vi "CreateCurveNamesvb.vi"(8 "error in":errorcluster, 9 "NomDon":string[](array[string])=["RTêta;", "X&Y;"], 10 "IndCourbe":i64 caption="Numéro de Balayage", 11 "Experiment.lvclass In":refnum<class "Experiment.lvclass">) -> (0 "error out":errorcluster, 2 "Scan list":string[](array[string]), 3 "Experiment.lvclass Out":refnum<class "Experiment.lvclass">, 4 "ScanTableSize":i32[](array[numeric]))   [LabVIEW 2019, in "Experiment.lvclass"]
doc: "Ce Vi créer la ligne d'entête du fichier texte de sauvegarde à partir du nombre de courbe voulu."
uses:
  Experiment.lvclass
  Experiment.lvclass/Experiment.ctl
  Calculations Class/Calculations.lvclass
  Calculations Class/Calculations.lvclass/Calculations.ctl
  Calculations Class/Accessor/GetCalcEveryScanPar.vi
  DevicesClass/BaseDevice/BaseDevice.lvclass
panel:
  out "CalcNameInd":i32[](array[numeric])
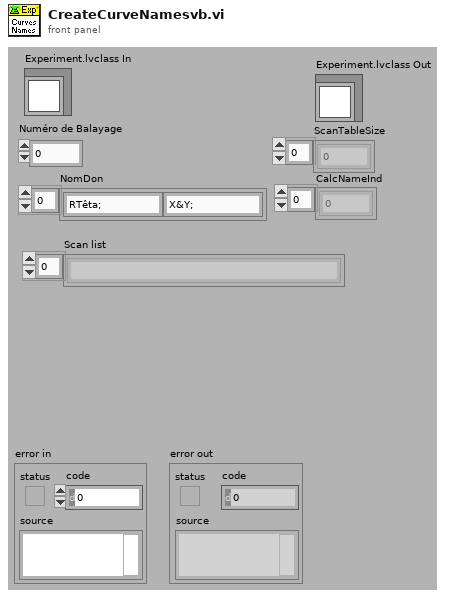
[diagram p1: front panel]
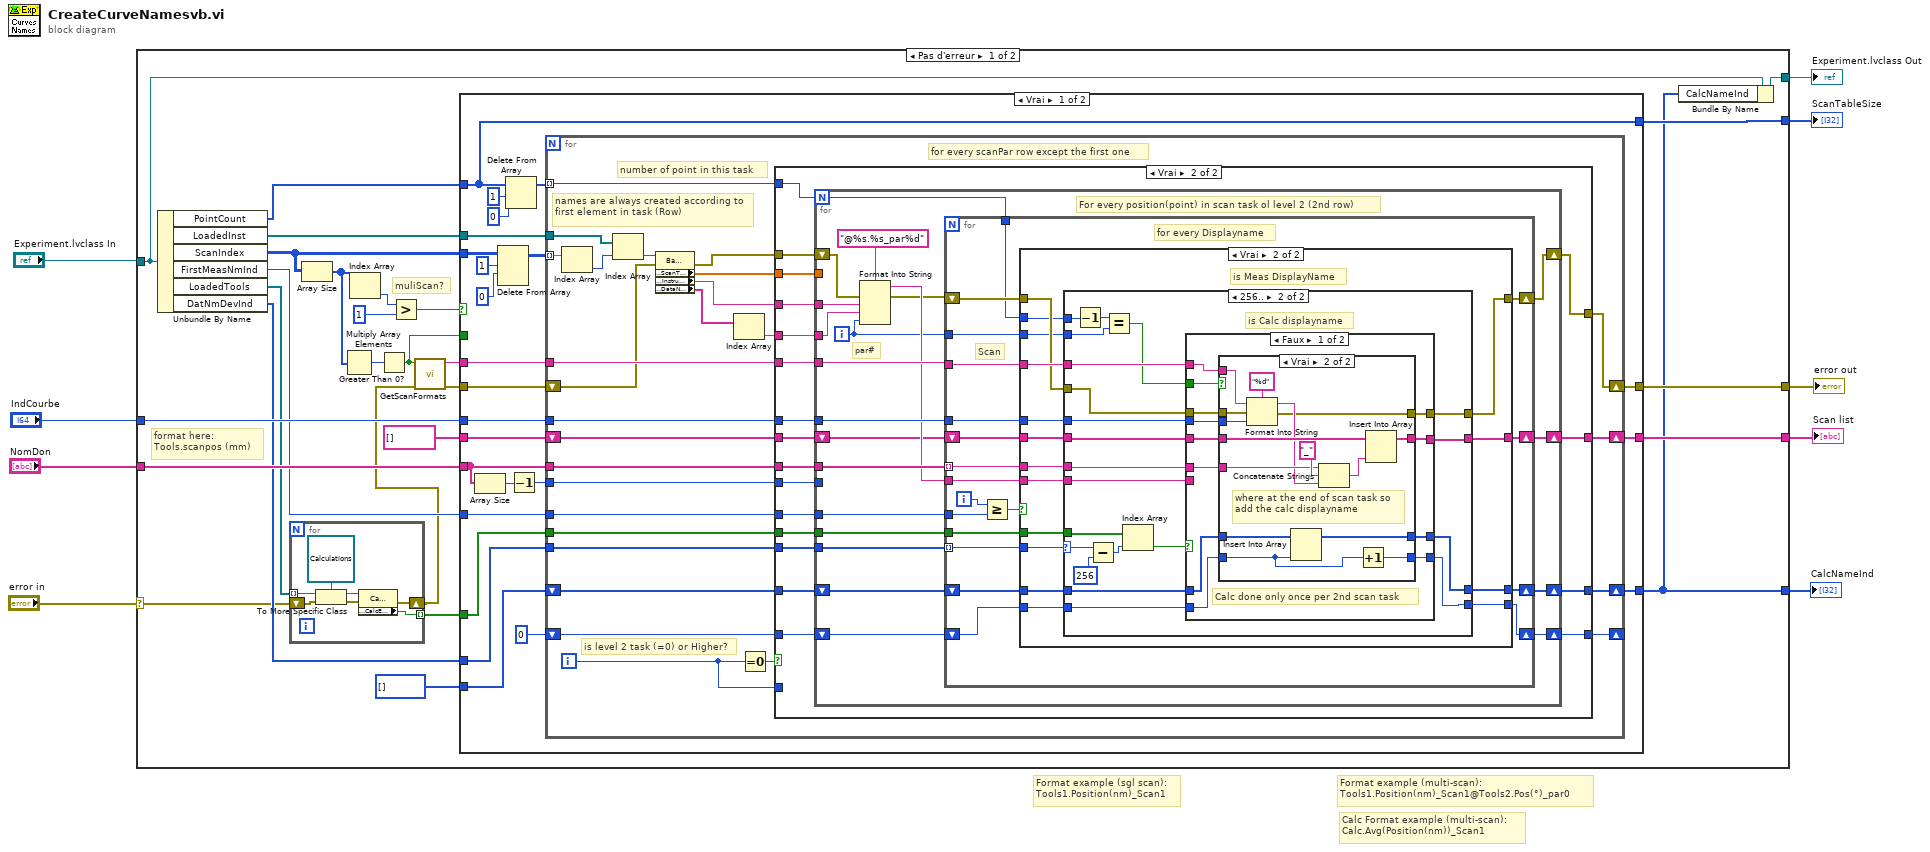
[diagram p0: block diagram]
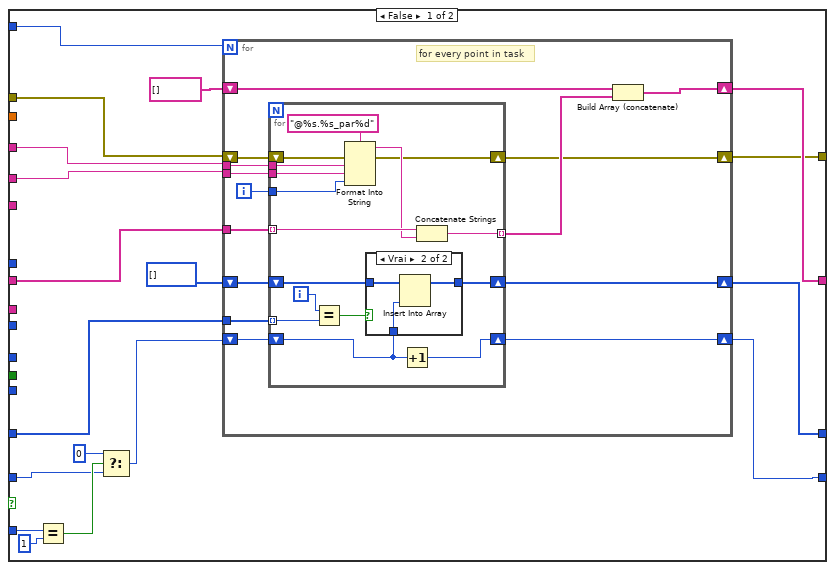
[diagram p2: hidden frame]
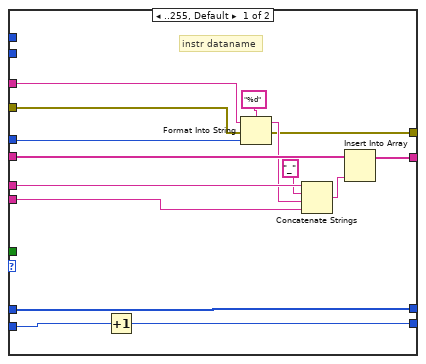
[diagram p5: hidden frame]
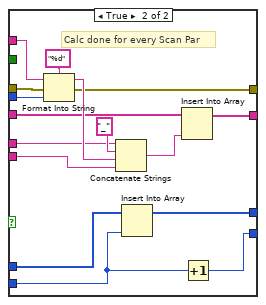
[diagram p7: hidden frame]
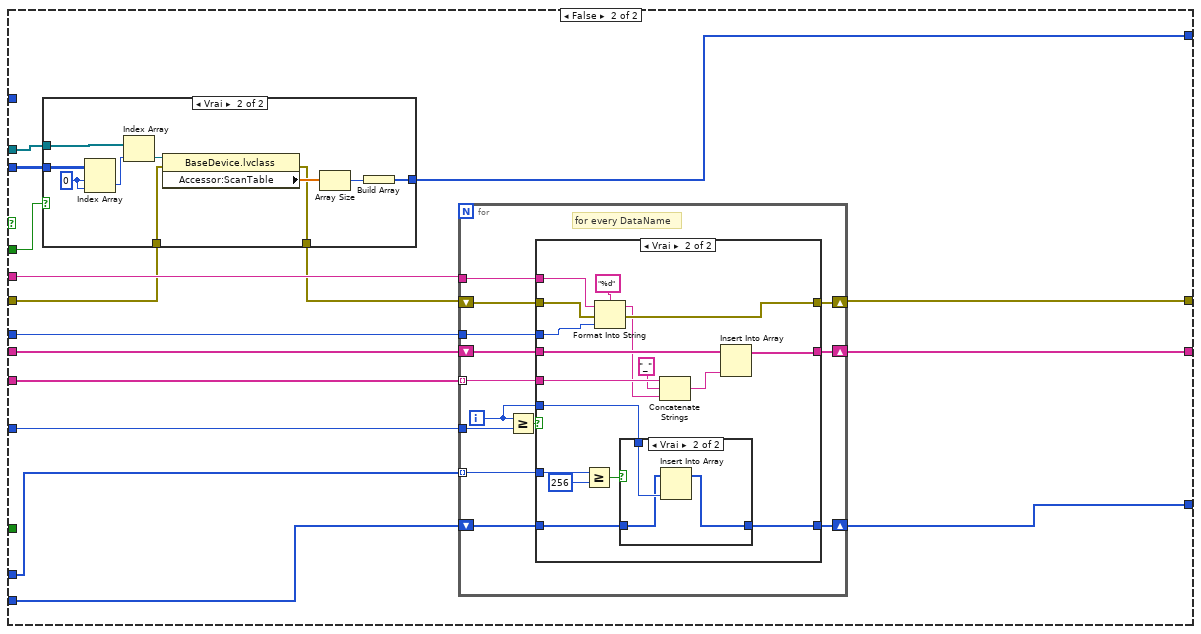
[diagram p8: hidden frame]
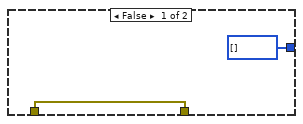
[diagram p9: hidden frame]
diagram:
  # "Calc Format example (multi-scan):\nCalc.Avg(Position(nm))_Scan1"
  # "Format example (multi-scan):\nTools1.Position(nm)_Scan1@Tools2.Pos(°)_par0"
  # "Format example (sgl scan):\nTools1.Position(nm)_Scan1"
  n1 = case shown="Pas d'erreur" "error in" {
    selector: "error in" -> [w15 w375]
    tunnel: [w26 w375] -> w8
    tunnel: [w32 _] -> w7
    tunnel: "NomDon" -> [w33 _]
    tunnel: "Experiment.lvclass In" -> [w23 w374]
    tunnel: "IndCourbe" -> [w35 _]
    tunnel: [w11 w374] -> w3
    tunnel: [w22 _] -> w2
    tunnel: [w10 _] -> w1
    frame No Error {
      # "format here:\nTools.scanpos (mm)"
      # "muliScan?"
      n2 = Unbundle By Name(w23) -> ("PointCount"=w18:i32[], "LoadedInst"=w27:refnum<class "BaseDevice.lvclass">[], "ScanIndex"=w28:i32[][], "FirstMeasNmInd"=w25:i32, "LoadedTools"=w16:refnum<class "BaseDevice.lvclass">[], "DatNmDevInd"=w17:i32[])
      n3 = for {
        tunnel: w16 -> [w40] mode=indexing
        shift-right: [w38] -> w14
        shift-left: w15 -> [w39]
        tunnel: [w37] -> w13 mode=indexing
        n4 = To More Specific Class(target class=refnum<class "Calculations.lvclass"> refnum ("Calculations.lvclass"), reference=w40, error in=w39) -> (specific class reference=w42:refnum<class "Calculations.lvclass">, error out=w43:errorcluster)
        n5 = property class="Calculations.lvclass"(reference=w42, error in=w43) -> (error out=w38:errorcluster, "Accessor:CalcEveryScanPar"=w37:bool)  [unwired: 1 out]
      }
      n6 = Array Size(array=w28) -> (size(s)=w20:i32[])
      n7 = Multiply Array Elements(1:w20) -> (0:w30:i32)
      n8 = Index Array(array=w20) -> (element=w19:i32)  [unwired: 1 in]
      n9 = Greater Than 0?(x=w30) -> (x > 0?=w21:bool)
      n10 = Greater?(x=w19, y=1) -> (0:w24:bool)
      n11 = call "GetScanFormats.vi"("ErrorIn(No Error)"=w14, "Scan(T)"=w21) -> ("sortie d'erreur"=w34:errorcluster, "Prefixe"=w36:string)  [unwired: 7 in, 1 out]
      n12 = case shown="Vrai" w24 {
        tunnel: w36 -> [w67 w324]
        tunnel: w35 -> [w66 w323]
        tunnel: w34 -> [w65 w314]
        tunnel: w33 -> [w51 w322]
        tunnel: [w60 w321] -> w32
        tunnel: string[] [] -> [w52 w320]
        tunnel: w28 -> [w64 w317]
        tunnel: w27 -> [w63 w316]
        tunnel: [w62 w319] -> w26
        tunnel: w25 -> [w61 w318]
        tunnel: [w47 w315] -> w22
        tunnel: w21 -> [_ w312]
        tunnel: w18 -> [w47 _]
        tunnel: w17 -> [w53 w310]
        tunnel: w13 -> [w48 _]
        tunnel: i32[] [] ("DatNameInd") -> [w46 w311]
        tunnel: [w44 w309] -> w10
        frame True {
          n13 = Array Size(array=w51) -> (size(s)=w50:i32)
          n14 = Delete From Array(array=w64, length=1 ("longueur"), index (row)=0 ("indice (ligne)")) -> (array with subset deleted=w59:i32[][])  [unwired: 1 in, 1 out]
          n15 = Delete From Array(array=w47, length=1 ("longueur"), index=0 ("indice")) -> (array with subset deleted=w55:i32[])  [unwired: 1 out]
          n16 = Decrement(x=w50) -> (x-1=w49:i32)
          n17 = for {
            tunnel: w67 -> [w94]
            tunnel: w66 -> [w93]
            tunnel: w51 -> [w92]
            tunnel: w59 -> [w91] mode=indexing
            tunnel: w63 -> [w90]
            shift-right: [w88] -> w62
            shift-left: w65 -> [w89]
            tunnel: w61 -> [w87]
            shift-right: [w84] -> w60
            shift-left: w52 -> [w83]
            tunnel: w55 -> [w82] mode=indexing
            tunnel: w53 -> [w75]
            tunnel: w48 -> [w74]
            tunnel: w49 -> [w73]
            shift-right: [w70] -> _
            shift-left: 0 ("Numérique") -> [w71]
            shift-right: [w69] -> w44
            shift-left: w46 -> [w72]
            i -> [w68]
            # "is level 2 task (=0) or Higher?"
            # "number of point in this task"
            # "names are always created according to first element in task (Row)"
            # "for every scanPar row except the first one"
            n18 = Index Array(array=w91) -> (element=w80:i32)  [unwired: 1 in]
            n19 = Index Array(array=w90, index=w80) -> (element=w79:refnum<class "BaseDevice.lvclass">)
            n20 = property class="BaseDevice.lvclass"(reference=w79, error in=w89) -> (error out=w81:errorcluster, "Accessor:ScanTable"=w77:dbl[], "Accessor:InstrumentName"=w85:string, "Accessor:DataNames"=w78:string[])  [unwired: 1 out]
            n21 = Index Array(array=w78) -> (element=w86:string)  [unwired: 1 in]
            n22 = Equal To 0?(x=w68) -> (x = 0?=w76:bool)
            n23 = case shown="Vrai" w76 {
              tunnel: w94 -> [_ w165]
              tunnel: w93 -> [_ w164]
              tunnel: w92 -> [_ w163]
              tunnel: [w107 w162] -> w88
              tunnel: w87 -> [_ w161]
              tunnel: w86 -> [w111 w160]
              tunnel: w85 -> [w112 w159]
              tunnel: [w108 w158] -> w84
              tunnel: w83 -> [w109 w157]
              tunnel: w82 -> [w105 w152]
              tunnel: w81 -> [w110 w156]
              tunnel: w77 -> [_ w155]
              tunnel: w75 -> [_ w154]
              tunnel: w74 -> [_ w153]
              tunnel: w73 -> [_ w151]
              tunnel: w72 -> [w101 w150]
              tunnel: w71 -> [w96 w149]
              tunnel: [w104 w148] -> w70
              tunnel: [w99 w147] -> w69
              tunnel: w68 -> [w103 _]
              frame False {
                n24 = Equal?(x=w103, y=1) -> (x = y?=w97:bool)
                n25 = Select(t=0, s=w97, f=w96) -> (s? t:f=w98:i32)
                n26 = for {
                  N: w105 -> [_]
                  tunnel: w112 -> [w126]
                  tunnel: w111 -> [w125]
                  shift-right: [w120] -> w107
                  shift-left: w110 -> [w124]
                  tunnel: w109 -> [w123]
                  shift-right: [w119] -> w108
                  shift-left: string[] [] -> [w118]
                  shift-right: [w117] -> w104
                  shift-left: w98 -> [w116]
                  tunnel: w101 -> [w115]
                  shift-right: [w113] -> w99
                  shift-left: i32[] [] ("DatNameInd") -> [w114]
                  i -> [w122]
                  # "for every point in task"
                  n27 = for {
                    tunnel: w126 -> [w141]
                    tunnel: w125 -> [w140]
                    tunnel: w123 -> [w138] mode=indexing
                    tunnel: w122 -> [w136]
                    tunnel: [w135] -> w121 mode=indexing
                    shift-right: [w134] -> w120
                    shift-left: w124 -> [w139]
                    shift-right: [w133] -> w117
                    shift-left: w116 -> [w127]
                    tunnel: w115 -> [w131] mode=indexing
                    shift-right: [w128] -> w113
                    shift-left: w114 -> [w129]
                    i -> [w130]
                    n28 = Equal?(x=w130, y=w131) -> (x = y?=w132:bool)
                    n29 = Format Into String(format string="@%s.%s_par%d" ("chaîne de format"), error in=w139, w141, w140, w136) -> (resulting string=w137:string, error out=w134:errorcluster)  [unwired: 1 in]
                    n30 = case shown="Vrai" w132 {
                      tunnel: w129 -> [w143 w146]
                      tunnel: [w143 w145] -> w128
                      tunnel: w127 -> [_ w144]
                      frame False {
                      }
                      frame True {
                        n31 = Insert Into Array(array=w146, new element=w144) -> (w145:i32[])  [unwired: 1 in]
                      }
                    }
                    n32 = Increment(x=w127) -> (x+1=w133:i32)
                    n33 = Concatenate Strings(w138, w137) -> (w135:string)
                  }
                  n34 = Build Array (concatenate)(w118, w121) -> (w119:string[])
                }
              }
              frame True {
                n35 = for {
                  N: w152 -> [w173]
                  tunnel: w165 -> [w186]
                  tunnel: w164 -> [w185]
                  tunnel: w163 -> [w184]
                  shift-right: [w170] -> w162
                  shift-left: w156 -> [w182]
                  tunnel: w161 -> [w183]
                  tunnel: w160 -> [w181]
                  tunnel: w159 -> [w180]
                  shift-right: [w171] -> w158
                  shift-left: w157 -> [w178]
                  tunnel: w155 -> [_]
                  tunnel: w154 -> [w175]
                  tunnel: w153 -> [w174]
                  tunnel: w151 -> [_]
                  shift-right: [w166] -> w147
                  shift-left: w150 -> [w169]
                  shift-right: [w167] -> w148
                  shift-left: w149 -> [w168]
                  i -> [w172]
                  # "par#"
                  # "For every position(point) in scan task ol level 2 (2nd row)"
                  n36 = Format Into String(format string="@%s.%s_par%d" ("chaîne de format"), error in=w182, w180, w181, w172) -> (resulting string=w179:string, error out=w177:errorcluster)  [unwired: 1 in]
                  n37 = for {
                    tunnel: w186 -> [w200]
                    tunnel: w184 -> [w203] mode=indexing
                    shift-right: [w204] -> w171
                    shift-left: w178 -> [w205]
                    tunnel: w185 -> [w201]
                    shift-right: [w191] -> w170
                    shift-left: w177 -> [w199]
                    tunnel: w183 -> [w198]
                    tunnel: w179 -> [w197]
                    tunnel: w175 -> [w196] mode=indexing
                    tunnel: w174 -> [w195]
                    tunnel: w173 -> [w193]
                    tunnel: w172 -> [w192]
                    shift-right: [w188] -> w166
                    shift-left: w169 -> [w189]
                    shift-right: [w187] -> w167
                    shift-left: w168 -> [w190]
                    i -> [w194]
                    # "Scan"
                    # "for every Displayname"
                    n38 = Greater Or Equal?(x=w194, y=w198) -> (x >= y?=w202:bool)
                    n39 = case shown="Vrai" w202 {
                      tunnel: w205 -> [w209 w225]
                      tunnel: [w209 w224] -> w204
                      tunnel: w203 -> [_ w223]
                      tunnel: w201 -> [_ w219]
                      tunnel: w200 -> [_ w222]
                      tunnel: w199 -> [w208 w221]
                      tunnel: w197 -> [_ w220]
                      tunnel: w196 -> [_ w217]
                      tunnel: w195 -> [_ w218]
                      tunnel: w193 -> [_ w216]
                      tunnel: w192 -> [_ w215]
                      tunnel: [w208 w214] -> w191
                      tunnel: w190 -> [w206 w213]
                      tunnel: w189 -> [w207 w212]
                      tunnel: [w207 w211] -> w188
                      tunnel: [w206 w210] -> w187
                      frame False {
                        # "in a scan the first items are the scanpar (var param): dont include it in graph legend"
                      }
                      frame True {
                        # "is Meas DisplayName"
                        n40 = case shown="256.." w217 {
                          selector: w217 -> [_ w252]
                          tunnel: w225 -> [w240 w258]
                          tunnel: [w239 w256] -> w224
                          tunnel: w223 -> [w238 w259]
                          tunnel: w222 -> [w237 w261]
                          tunnel: w221 -> [w236 w246]
                          tunnel: w220 -> [w232 w257]
                          tunnel: w219 -> [w231 w260]
                          tunnel: w218 -> [_ w255]
                          tunnel: w216 -> [_ w251]
                          tunnel: w215 -> [_ w249]
                          tunnel: [w229 w247] -> w214
                          tunnel: w213 -> [w227 w244]
                          tunnel: w212 -> [w228 w243]
                          tunnel: [w228 w242] -> w211
                          tunnel: [w226 w241] -> w210
                          frame ..255, Default {
                            # "instr dataname"
                            n41 = Increment(x=w227) -> (x+1=w226:i32)
                            n42 = Format Into String(format string="%d" ("chaîne de format"), initial string=w237, error in=w236, w231) -> (resulting string=w234:string, error out=w229:errorcluster)
                            n43 = Concatenate Strings(w238, "_" ("chaîne"), w234, w232) -> (w235:string)
                            n44 = Insert Into Array(array=w240, new element=w235) -> (w239:string[])  [unwired: 1 in]
                          }
                          frame 256.. {
                            # "is Calc displayname"
                            n45 = Decrement(x=w251) -> (x-1=w250:i32)
                            n46 = Subtract(x=w252, y=256) -> (x-y=w254:i32)
                            n47 = Equal?(x=w250, y=w249) -> (x = y?=w248:bool)
                            n48 = Index Array(array=w255, index=w254) -> (element=w245:bool)
                            n49 = case shown="Faux" w245 {
                              tunnel: w261 -> [w269 w304]
                              tunnel: w260 -> [w273 w303]
                              tunnel: w259 -> [w271 w302]
                              tunnel: w258 -> [w272 w301]
                              tunnel: w257 -> [_ w299]
                              tunnel: [w270 w300] -> w256
                              tunnel: w248 -> [w268 _]
                              tunnel: [w267 w298] -> w247
                              tunnel: w246 -> [w266 w297]
                              tunnel: w244 -> [w264 w294]
                              tunnel: w243 -> [w265 w296]
                              tunnel: [w263 w295] -> w242
                              tunnel: [w262 w293] -> w241
                              frame False {
                                # "Calc done only once per 2nd scan task"
                                n50 = case shown="Vrai" w268 {
                                tunnel: w269 -> [_ w291]
                                tunnel: w273 -> [_ w290]
                                tunnel: w272 -> [w277 w287]
                                tunnel: w271 -> [_ w286]
                                tunnel: [w277 w284] -> w270
                                tunnel: [w276 w283] -> w267
                                tunnel: w266 -> [w276 w282]
                                tunnel: w265 -> [w275 w281]
                                tunnel: w264 -> [w274 w279]
                                tunnel: [w275 w280] -> w263
                                tunnel: [w274 w278] -> w262
                                frame False {
                                }
                                frame True {
                                # "where at the end of scan task so add the calc displayname"
                                n51 = Format Into String(format string="%d" ("chaîne de format"), initial string=w291, error in=w282, w290) -> (resulting string=w285:string, error out=w283:errorcluster)
                                n52 = Insert Into Array(array=w281, new element=w279) -> (w280:i32[])  [unwired: 1 in]
                                n53 = Concatenate Strings(w286, "_" ("chaîne"), w285) -> (w288:string)
                                n54 = Increment(x=w279) -> (x+1=w278:i32)
                                n55 = Insert Into Array(array=w287, new element=w288) -> (w284:string[])  [unwired: 1 in]
                                }
                                }
                              }
                              frame True {
                                # "Calc done for every Scan Par"
                                n56 = Format Into String(format string="%d" ("chaîne de format"), initial string=w304, error in=w297, w303) -> (resulting string=w306:string, error out=w298:errorcluster)
                                n57 = Concatenate Strings(w302, "_" ("chaîne"), w306, w299) -> (w305:string)
                                n58 = Insert Into Array(array=w296, new element=w294) -> (w295:i32[])  [unwired: 1 in]
                                n59 = Insert Into Array(array=w301, new element=w305) -> (w300:string[])  [unwired: 1 in]
                                n60 = Increment(x=w294) -> (x+1=w293:i32)
                              }
                            }
                          }
                        }
                      }
                    }
                  }
                }
              }
            }
          }
        }
        frame False {
          n61 = case shown="Vrai" w312 {
            tunnel: w317 -> [_ w334]
            tunnel: w316 -> [_ w332]
            tunnel: [i32[] [] w329] -> w315
            tunnel: w314 -> [w326 w328]
            tunnel: [w326 w327] -> w313
            frame False {
            }
            frame True {
              w333 = 0 ("indice (ligne)")
              n62 = Index Array(array=w334, index (row)=w333, index (col)=w333) -> (element=w336:i32)
              n63 = Index Array(array=w332, index=w336) -> (element=w335:refnum<class "BaseDevice.lvclass">)
              n64 = property class="BaseDevice.lvclass"(reference=w335, error in=w328) -> (error out=w327:errorcluster, "Accessor:ScanTable"=w331:dbl[])  [unwired: 1 out]
              n65 = Array Size(array=w331) -> (size(s)=w330:i32)
              n66 = Build Array(w330) -> (w329:i32[])
            }
          }
          n67 = for {
            tunnel: w324 -> [w344]
            tunnel: w322 -> [w347] mode=indexing
            shift-right: [w348] -> w321
            shift-left: w320 -> [w349]
            tunnel: w323 -> [w345]
            shift-right: [w342] -> w319
            shift-left: w313 -> [w343]
            tunnel: w318 -> [w341]
            shift-right: [w338] -> w309
            shift-left: w311 -> [w339]
            tunnel: w310 -> [w337] mode=indexing
            i -> [w340]
            # "for every DataName"
            n68 = Greater Or Equal?(x=w340, y=w341) -> (x >= y?=w346:bool)
            n69 = case shown="Vrai" w346 {
              tunnel: w349 -> [w352 w369]
              tunnel: [w352 w368] -> w348
              tunnel: w347 -> [_ w367]
              tunnel: w345 -> [_ w360]
              tunnel: w344 -> [_ w366]
              tunnel: w343 -> [w351 w365]
              tunnel: [w351 w364] -> w342
              tunnel: w340 -> [_ w358]
              tunnel: w339 -> [w350 w357]
              tunnel: [w350 w356] -> w338
              tunnel: w337 -> [_ w355]
              frame False {
                # "in a scan the first items are the scanpar (var param): dont include it in graph legend"
              }
              frame True {
                n70 = Greater Or Equal?(x=w355, y=256) -> (x >= y?=w353:bool)
                n71 = Format Into String(format string="%d" ("chaîne de format"), initial string=w366, error in=w365, w360) -> (resulting string=w362:string, error out=w364:errorcluster)
                n72 = case shown="Vrai" w353 {
                  tunnel: w358 -> [_ w373]
                  tunnel: w357 -> [w370 w372]
                  tunnel: [w370 w371] -> w356
                  frame False {
                  }
                  frame True {
                    n73 = Insert Into Array(array=w372, new element=w373) -> (w371:i32[])  [unwired: 1 in]
                  }
                }
                n74 = Concatenate Strings(w367, "_" ("chaîne"), w362) -> (w363:string)
                n75 = Insert Into Array(array=w369, new element=w363) -> (w368:string[])  [unwired: 1 in]
              }
            }
          }
        }
      }
      n76 = Bundle By Name(cluster=w23, "CalcNameInd"=w10) -> (w11:refnum<class "Experiment.lvclass">)
    }
    frame Error {
    }
  }
  "error out" <- w8
  "Scan list" <- w7
  "Experiment.lvclass Out" <- w3
  "ScanTableSize" <- w2
  "CalcNameInd" <- w1
